vi "Drive_AutoShift (3).vi"(5 "Max":dbl format="%#_13g", 6 "Force Low Gear":bool, 7 "ShifterRef":T2={"DevStatus"={"status"=FALSE, "code"=0, "source"=""}, "Pneumatics Control Module"=0, "Forward Solenoid Channel"=enum."Invalid", "Reverse Solenoid Channel"=enum."Invalid"}, 8 "Right  Input":dbl, 9 "Left Input":dbl, 10 "Right RPM":dbl, 11 "Left RPM":dbl) -> (1 "Shifting":bool, 2 "Right Output":dbl, 3 "Left Output":dbl, 4 "Gear":T1)   [LabVIEW 2016]
uses:
  <vilib>/Rock Robotics/WPI/Solenoid/WPI_SolenoidDevRef.ctl
  <vilib>/Rock Robotics/WPI/Solenoid/WPI_SolenoidChannel.ctl
  <vilib>/Rock Robotics/WPI/Solenoid/WPI_SolenoidValue.ctl
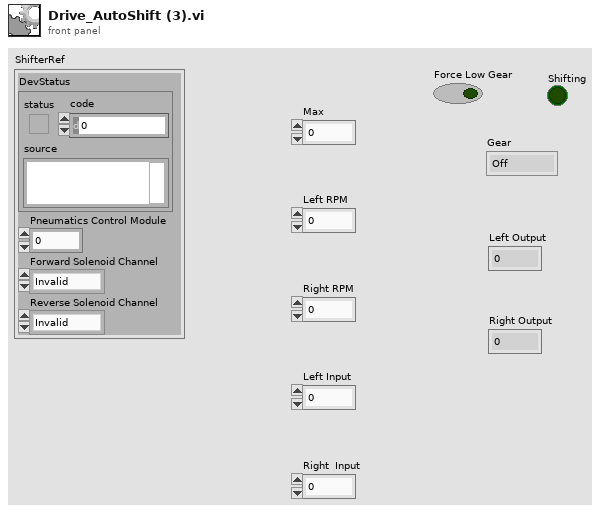
[diagram p1: front panel]
types:
  T1 = typedef "WPI_SolenoidValue.ctl" = enum16{"Off", "On", "Forward", "Reverse"}
  T2 = typedef "WPI_SolenoidDevRef.ctl" = cluster{"DevStatus":errorcluster, "Pneumatics Control Module":u8, "Forward Solenoid Channel":T3, "Reverse Solenoid Channel":T3}
  T3 = typedef "WPI_SolenoidChannel.ctl" = enum8{"Solenoid 0", "Solenoid 1", "Solenoid 2", "Solenoid 3", "Solenoid 4", "Solenoid 5", "Solenoid 6", "Solenoid 7", "Invalid"}
  T4 = cluster{"OutputMAX":dbl, "OutputMIN":dbl, "InputMAX":dbl, "InputMIN":dbl}
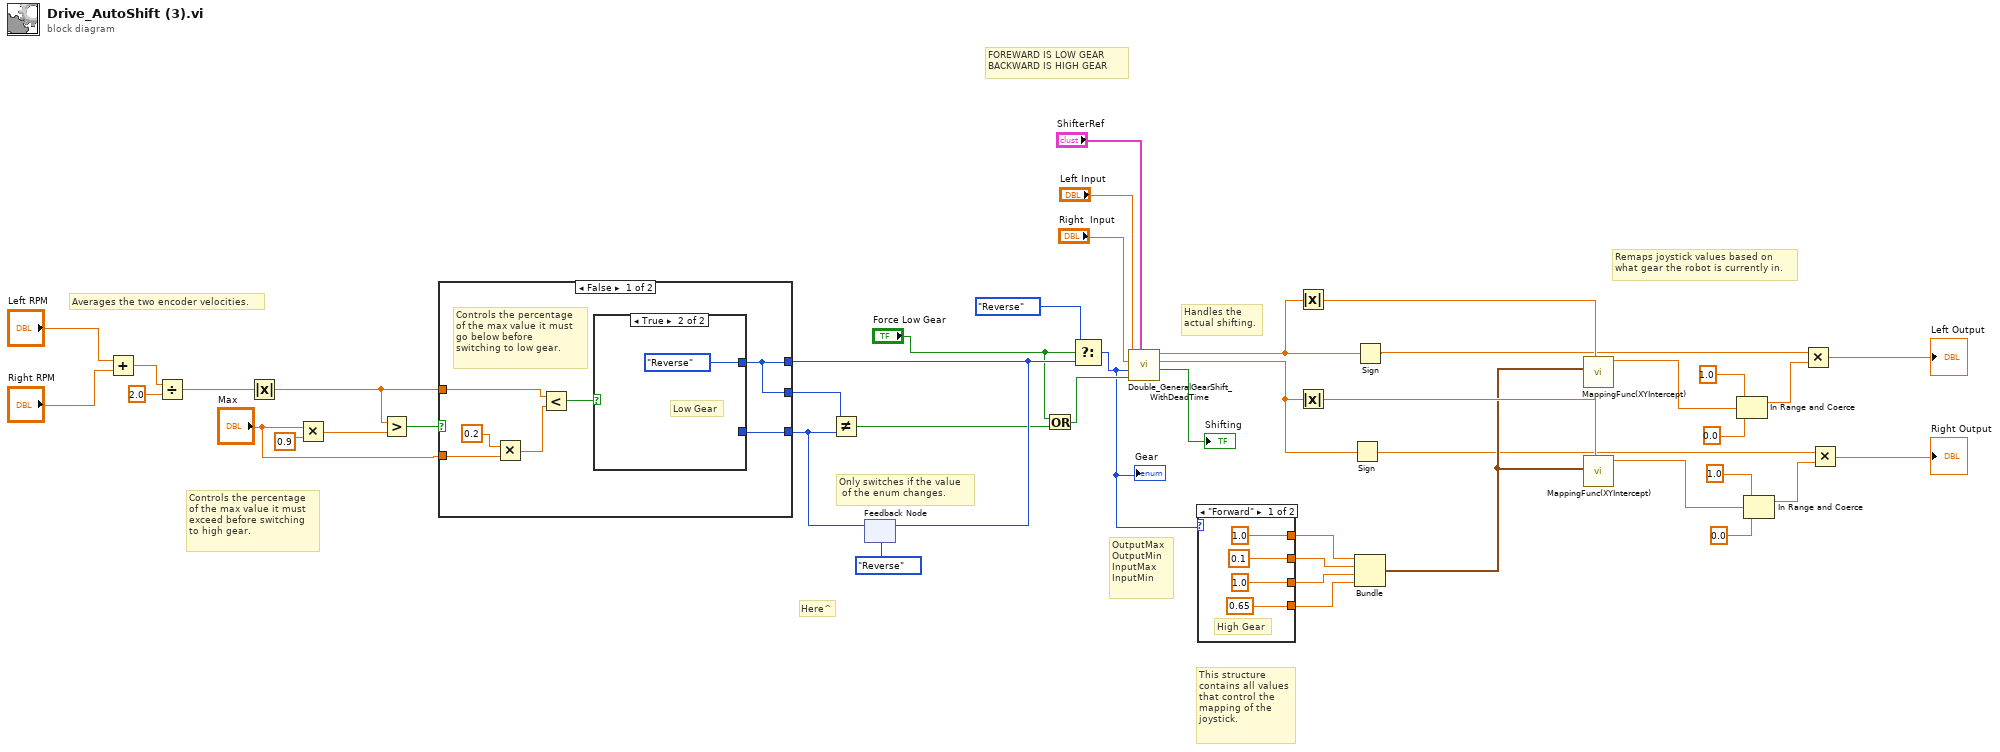
[diagram p0: block diagram]
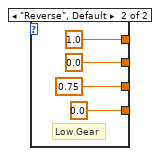
[diagram p2: hidden frame]
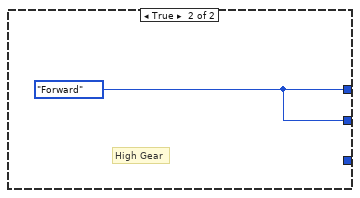
[diagram p4: hidden frame]
diagram:
  # "Here^"
  # "OutputMax\nOutputMin\nInputMax\nInputMin"
  # "This structure\ncontains all values\nthat control the\nmapping of the \njoystick."
  # "Remaps joystick values based on\nwhat gear the robot is currently in."
  # "Handles the\nactual shifting."
  # "FOREWARD IS LOW GEAR\nBACKWARD IS HIGH GEAR"
  # "Only switches if the value\n of the enum changes."
  # "Controls the percentage\nof the max value it must \nexceed before switching\nto high gear."
  # "Averages the two encoder velocities."
  n1 = Add(x="Left RPM", y="Right RPM") -> (x+y=w31:dbl)
  n2 = Divide(x=w31, y=2.0) -> (x/y=w7:dbl)
  n3 = Absolute Value(x=w7) -> (abs(x)=w6:dbl)
  n4 = Multiply(x="Max", y=0.9) -> (x*y=w43:dbl)
  n5 = Greater?(x=w6, y=w43) -> (0:w42:bool)
  n6 = feedback #1(WPI_SolenoidValue."Reverse" ("Shift Value")) -> (w40:T1)
  n7 = case shown="False" w42 {
    tunnel: [w47 w54] -> w21
    tunnel: [w47 w54] -> w41
    tunnel: "Max" -> [w50 _]
    tunnel: w40 -> [w46 _]
    tunnel: w6 -> [w45 _]
    frame False {
      # "Controls the percentage\nof the max value it must \ngo below before \nswitching to low gear."
      n8 = Multiply(x=0.2, y=w50) -> (x*y=w48:dbl)
      n9 = Less?(x=w45, y=w48) -> (x < y?=w51:bool)
      n10 = case shown="True" w51 {
        tunnel: [w52 WPI_SolenoidValue."Reverse" ("Shift Value")] -> w47
        tunnel: w46 -> [w52 _]
        frame False {
        }
        frame True {
          # "Low Gear"
        }
      }
    }
    frame True {
      w54 = WPI_SolenoidValue."Forward" ("Shift Value")
      # "High Gear"
    }
  }
  n11 = Not Equal?(x=w41, y=w40) -> (x != y?=w5:bool)
  n12 = feedback-in #1(w21) -> ()
  n13 = Or(x="Force Low Gear", y=w5) -> (x .or. y?=w4:bool)
  n14 = Select(t=WPI_SolenoidValue."Reverse", s="Force Low Gear", f=w21) -> (s? t:f=w3:T1)
  "Gear" <- w3
  n15 = call "Double_GeneralGearShift_WithDeadTime.vi"("ShifterRef"="ShifterRef", "Shift Control"=w4, "Shift Value"=w3, "Right"="Right  Input", "Left"="Left Input") -> ("Shifting"=→"Shifting":bool, "Right Output"=w15:dbl, "Left Output"=w13:dbl)  [unwired: 3 in, 1 out]
  n16 = case shown="\"Forward\"" w3 {
    tunnel: [1.0 ("OutputMAX") 1.0 ("OutputMAX")] -> w18
    tunnel: [0.1 ("OutputMIN") 0.0 ("OutputMIN")] -> w17
    tunnel: [1.0 ("InputMAX") 0.75 ("InputMAX")] -> w19
    tunnel: [0.65 ("InputMIN") 0.0 ("InputMIN")] -> w20
    frame "Forward" {
      # "High Gear"
    }
    frame "Reverse", Default {
      # "Low Gear"
    }
  }
  n17 = Absolute Value(x=w13) -> (abs(x)=w36:dbl)
  n18 = Absolute Value(x=w15) -> (abs(x)=w26:dbl)
  n19 = Sign(1:w15) -> (0:w14:dbl)
  n20 = Sign(1:w13) -> (0:w12:dbl)
  n21 = Bundle("OutputMAX"=w18, "OutputMIN"=w17, "InputMAX"=w19, "InputMIN"=w20) -> (w16:T4)  [unwired: 1 in]
  n22 = call "MappingFunc(XYIntercept).vi"("Input"=w36, "Cluster"=w16) -> ("Output"=w35:dbl)  [unwired: 9 in]
  n23 = call "MappingFunc(XYIntercept).vi"("Input"=w26, "Cluster"=w16) -> ("Output"=w27:dbl)  [unwired: 9 in]
  n24 = In Range and Coerce(upper limit=1.0, x=w35, lower limit=0.0) -> (coerced(x)=w32:dbl)  [unwired: 1 out]
  n25 = In Range and Coerce(upper limit=1.0, x=w27, lower limit=0.0) -> (coerced(x)=w28:dbl)  [unwired: 1 out]
  n26 = Multiply(x=w12, y=w32) -> (x*y=→"Left Output":dbl)
  n27 = Multiply(x=w14, y=w28) -> (x*y=→"Right Output":dbl)
